vi "TextColor.vi"(8 "valueStatus":T1, 10 "reference":refnum<vi>) -> ()   [LabVIEW 2014, in "Panels.lvlib"]
uses:
  Panels.lvlib
  CSlibraries/UtilityLib/UtilityLib.lvlib
  CSlibraries/UtilityLib/UtilityLib.valueStatus.ctl
panel:
  in  "error in (no error)":errorcluster
  out "error out":errorcluster
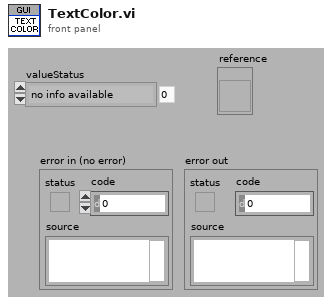
[diagram p1: front panel]
types:
  T1 = typedef "UtilityLib.lvlib/UtilityLib.valueStatus.ctl" = enum16{"no info available", "stand by/off", "on", "warning", "alarm/malfunction", "not implemented", "user action required", "important information", "system default", "control default", "indicator default", "button default"}
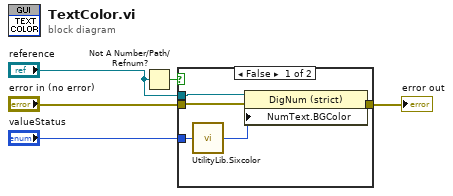
[diagram p0: block diagram]
diagram:
  n1 = Not A Number/Path/Refnum?(number/path/refnum="reference") -> (NaN/Path/Refnum?=w3:bool)
  n2 = case shown="False" w3 {
    tunnel: "reference" -> [w8 _]
    tunnel: "error in (no error)" -> [w7 w11]
    tunnel: [w9 w11] -> w5
    tunnel: "valueStatus" -> [w10 _]
    frame False {
      n3 = call "UtilityLib.Sixcolor.vi"("State"=w10) -> ("Color Box"=w6:u32)
      n4 = property on="Property Node" class="DigNum (strict)"(reference=w8, error in=w7, "NumText.BGColor"=w6) -> (error out=w9:errorcluster)  [unwired: 1 out]
    }
    frame True {
    }
  }
  "error out" <- w5
